vi "DriveExecute_PID_Autotune.vi"(8 "error in (no error)":errorcluster) -> (0 "error out":errorcluster)   [LabVIEW 2020]
doc: "Execute for Drie\n\nClosed control loop for drive\n\ninput: \n error in (cluster)\n\noutput:\n error out (cluster)"
uses:
  <vilib>/Rock Robotics/WPI/ThirdParty/Phoenix-LabVIEW/Motor Controller/Controls/CTRE_Phoenix_MotorControl_ControlMode.ctl
  <vilib>/Rock Robotics/WPI/ThirdParty/JAS_Junk/TrajLib/SimpleMotorFF_Calculate.vi
  <vilib>/Rock Robotics/WPI/ThirdParty/JAS_Junk/TrajLib/VI/Util_GetTime_U32.vi
  <vilib>/Rock Robotics/WPI/ThirdParty/JAS_Junk/TrajLib/PIDController_AtSetpoint.vi
  <vilib>/Rock Robotics/WPI/ThirdParty/JAS_Junk/TrajLib/PIDController_SetPIDF.vi
  <vilib>/Rock Robotics/WPI/ThirdParty/JAS_Junk/TrajLib/PIDController_SetDerivativeFilter.vi
  <vilib>/Rock Robotics/WPI/ThirdParty/JAS_Junk/TrajLib/PIDController_SetIntegratorRange.vi
  <vilib>/Rock Robotics/WPI/ThirdParty/JAS_Junk/TrajLib/PIDController_SetTolerancePandV.vi
  <vilib>/Rock Robotics/WPI/ThirdParty/JAS_Junk/TrajLib/PIDController_DisableContinousInput.vi
  <vilib>/Rock Robotics/WPI/ThirdParty/JAS_Junk/TrajLib/PIDController_EnableContinousInput.vi
  <vilib>/Rock Robotics/WPI/ThirdParty/JAS_Junk/TrajLib/PIDController_Reset.vi
  <vilib>/Rock Robotics/WPI/ThirdParty/JAS_Junk/TrajLib/PIDController_New.vi
  <vilib>/Rock Robotics/WPI/ThirdParty/JAS_Junk/TrajLib/PIDController_SetOutputLimits.vi
  <vilib>/Rock Robotics/WPI/ThirdParty/JAS_Junk/TrajLib/SlewRateLimiter_New.vi
  <vilib>/Rock Robotics/WPI/ThirdParty/JAS_Junk/TrajLib/SlewRateLimiter_Reset.vi
  <vilib>/Rock Robotics/WPI/ThirdParty/JAS_Junk/TrajLib/SlewRateLimiter_Calculate.vi
  <vilib>/Rock Robotics/WPI/ThirdParty/JAS_Junk/TrajLib/SlewRateLimiter_SetRate.vi
  <vilib>/Rock Robotics/WPI/ThirdParty/JAS_Junk/TrajLib/LinearFilter_ResetToValue.vi
  <vilib>/Rock Robotics/WPI/ThirdParty/JAS_Junk/TrajLib/LinearFilter_Calculate.vi
  <vilib>/Rock Robotics/WPI/ThirdParty/JAS_Junk/TrajLib/PIDController_NewPeriod.vi
  <vilib>/Rock Robotics/SystemInterfaces/NetworkCommunication/NetComm_UsageReport_report.vi
  <vilib>/Rock Robotics/SystemInterfaces/Utilities/FPGA_UtilitiesRead LocalTime.vi
  <vilib>/Rock Robotics/WPI/ThirdParty/JAS_Junk/TrajLib/VI/Util_GetTime_U64.vi
  DriveGlobal.vi
  <vilib>/Rock Robotics/WPI/ThirdParty/JAS_Junk/TrajLib/LinearFilter_MovingAverage.vi
  <vilib>/Rock Robotics/WPI/ThirdParty/JAS_Junk/TrajLib/LinearFilter_LowPassBW1.vi
  <vilib>/Rock Robotics/WPI/ThirdParty/JAS_Junk/TrajLib/LinearFilter_LowPassBW2.vi
  <vilib>/Rock Robotics/WPI/ThirdParty/JAS_Junk/TrajLib/LinearFilter_HighPassBW1.vi
  <vilib>/Rock Robotics/WPI/ThirdParty/JAS_Junk/TrajLib/LinearFilter_HighPassBW2.vi
  <vilib>/Rock Robotics/WPI/ThirdParty/JAS_Junk/TrajLib/Globals/Util_LibraryGlobals.vi
  <vilib>/Rock Robotics/WPI/ThirdParty/JAS_Junk/TrajLib/PIDController_AdvCalculate_FF_Sp_Pv.vi
  <vilib>/Rock Robotics/Network Tables/NT Write Value.vi
  <vilib>/Rock Robotics/Network Tables/NT Write Boolean.vi
  <vilib>/Rock Robotics/Network Tables/NT Write Number.vi
  <vilib>/Rock Robotics/WPI/ThirdParty/JAS_Junk/TrajLib/Trajectory_Library.lvlib
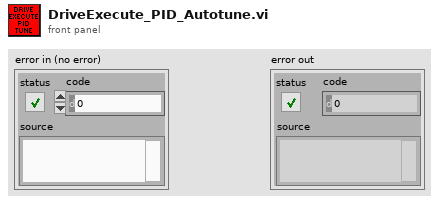
[diagram p1: front panel]
types:
  T1 = enum16{"Moving Average", "Low Pass 1st Order Butterworth", "Low Pass 2nd Order Butterworth", "High Pass 1st Order Butterworth", "High Pass 2nd Order Butterworth"}
  T2 = enum16{"Ziegler Nicols - Fast", "Ziegler Nicols - Normal", "Ziegler Nicols - Slow", "CHR regulator - 0% overshoot", "CHR regulator - 20% overshoot", "CHR servo - 0 % overshoot", "CHR servo - 20% overshoot"}
  T3 = typedef "CTRE_Phoenix_MotorControl_ControlMode.ctl" = u16
  T4 = typedef "WPI_EncoderDevRef.ctl" = cluster{"DevStatus":errorcluster, "EncoderIndex":T5, "CounterIndex":T6, "DistancePerCount":dbl, "Decoding Type":T7}
  T5 = typedef "FPGA_EncoderIdx.ctl" = enum8{"Enc 0", "Enc 1", "Enc 2", "Enc 3", "Enc 4", "Enc 5", "Enc 6", "Enc 7", "Invalid"}
  T6 = typedef "FPGA_CounterCtrSystemIndex.ctl" = enum8{"Ctr 0", "Ctr 1", "Ctr 2", "Ctr 3", "Ctr 4", "Ctr 5", "Ctr 6", "Ctr 7", "Invalid"}
  T7 = typedef "WPI_EncoderType.ctl" = enum16{"1x", "2x", "4x"}
  T8 = typedef "WPI_MotorControlDeviceRef.ctl" = cluster{"DeviceStatus":errorcluster, "Type":T9, "PWM":cluster{"PWM Channel":T10, "DeadBand":T11}, "CAN":cluster{"Device Number":u8, "SetOutput VI Ref":variant, "GetOutput VI Ref":variant, "Enable VI Ref":variant, "Disable VI Ref":variant, "Data":variant}, "Invert":bool, "DIO PWM":cluster{"PWM \"Enable\" Channel":T10, "DIOChannel":T12, "PWM Rate":dbl}}
  T9 = typedef "WPI_MotorControlType.ctl" = enum16{"PWM", "CAN", "DIO PWM"}
  T10 = typedef "FPGA_DIOPWMChannel.ctl" = enum8{"PWM 0", "PWM 1", "PWM 2", "PWM 3", "PWM 4", "PWM 5", "PWM 6", "PWM 7", "PWM 8", "PWM 9", "PWM MXP 0", "PWM MXP 1", "PWM MXP 2", "PWM MXP 3", "PWM MXP 4", "PWM MXP 5", "PWM MXP 6", "PWM MXP 7", "PWM MXP 8", "PWM MXP 9", "Invalid"}
  T11 = typedef "WPI_PWMDeadband.ctl" = cluster{"Name":string, "maxPositivePwm":i32, "minPositivePwm":i32, "centerPwm":i32, "maxNegativePwm":i32, "minNegativePwm":i32, "angularRange":u16}
  T12 = typedef "FPGA_DIOChannel.ctl" = enum8{"DIO 0", "DIO 1", "DIO 2", "DIO 3", "DIO 4", "DIO 5", "DIO 6", "DIO 7", "DIO 8", "DIO 9", "DIO MXP 0", "DIO MXP 1", "DIO MXP 2", "DIO MXP 3", "DIO MXP 4", "DIO MXP 5", "DIO MXP 6", "DIO MXP 7", "DIO MXP 8", "DIO MXP 9", "DIO MXP 10", "DIO MXP 11", "DIO MXP 12", "DIO MXP 13", "DIO MXP 14", "DIO MXP 15", "SPI Port CS1", "SPI Port CS2", "SPI Port CS3", "SPI Port MISO", "SPI Port MOSI", "Invalid"}
  T13 = typedef "ADIS16470 Device Reference.ctl" = cluster{"DevStatus":errorcluster, "Hardware Config":T14, "Calibration Complete":refnum<notifier>, "Status Reference":refnum<data-value>, "Data Reference":refnum<data-value>, "Sychronous Process VI":T17, "Cmd FIFO":refnum<k33>, "Source":T18, "Data FIFO":refnum<k33>, "Calibration Time (ms)":u32, "Data Reference":refnum<data-value>}
  T14 = typedef "ADIS16470 Hardware Configuration.ctl" = cluster{"SPI Clock Rate (Hz)":dbl, "IMU SPI Mode (3)":T15, "IMU Reset Pin":T12, "IMU SPI Bus":T16, "IMU Data Ready Pin":T12, "Stall Config":cluster{"Pow2BytesPerRead":u8, "StallTicks":u16, "CsToSclkTicks":u8}}
  T15 = typedef "WPI_SPIMode.ctl" = enum16{"Mode 0 (Clk Idle Low,Sample on Leading)", "Mode 1 (Clk Idle Low,Sample on Trailing)", "Mode 2 (Clk Idle High,Sample on Leading)", "Mode 3 (Clk Idle High,Sample on Trailing)"}
  T16 = typedef "spi_bus.ctl" = enum16{"SPI On-Board, CS0", "SPI On-Board, CS1", "SPI On-Board, CS2", "SPI On-Board, CS3", "SPI MXP", "Invalid"}
  T17 = typedef "ADIS16470 Process.ctl" = refnum<vi>
  T18 = typedef "FPGA_CounterEncoderSourceConvertionLVSourceType.ctl" = cluster{"DevStatus":errorcluster, "AnalogTriggerMode?":bool, "DigitalMode":cluster{"DIO Channel":T19}, "AnalogTriggerMode":cluster{"AnalogTriggerIndex":T20, "OutputType":T21}}
  T19 = typedef "FPGA_DIODigitalSourceChannel.ctl" = enum8{"DIO 0", "DIO 1", "DIO 2", "DIO 3", "DIO 4", "DIO 5", "DIO 6", "DIO 7", "DIO 8", "DIO 9", "DIO MXP 0", "DIO MXP 1", "DIO MXP 2", "DIO MXP 3", "DIO MXP 4", "DIO MXP 5", "DIO MXP 6", "DIO MXP 7", "DIO MXP 8", "DIO MXP 9", "DIO MXP 10", "DIO MXP 11", "DIO MXP 12", "DIO MXP 13", "DIO MXP 14", "DIO MXP 15", "SPI Port CS1", "SPI Port CS2", "SPI Port CS3", "SPI Port MISO", "SPI Port MOSI", "Disabled"}
  T20 = typedef "FPGA_AnalogTriggerIndex.ctl" = enum8{"Trig 0", "Trig 1", "Trig 2", "Trig 3", "Trig 4", "Trig 5", "Trig 6", "Trig 7", "Invalid"}
  T21 = typedef "FPGA_AnalogTriggerOutType.ctl" = enum16{"InWindow", "TriggerState", "Rising", "Falling"}
  T22 = typedef "ADIS16470 Data.ctl" = cluster{"XAngle":dbl, "YAngle":dbl, "ZAngle":dbl}
  T23 = typedef "Trajectory_Library.lvlib/SIMPLE_MOTOR_FF.ctl" = cluster{"Ks":dbl, "Kv":dbl, "Ka":dbl, "KnInv":dbl}
  T24 = typedef "Trajectory_Library.lvlib/PID_ADV_LIMITS.ctl" = cluster{"MaxInput":dbl, "MinInput":dbl, "Continuous":bool, "MaxOutput":dbl, "MinOutput":dbl}
  T25 = typedef "Trajectory_Library.lvlib/PID_ADV_TUNING.ctl" = cluster{"Kf":dbl, "Kp":dbl, "Ki":dbl, "Kd":dbl, "MaximumIntegral":dbl, "MinimumIntegral":dbl, "Filter Derivative":bool}
  T26 = cluster{"Controller Constant Type":enum16{"Ziegler Nicols - Fast", "Ziegler Nicols - Normal", "Ziegler Nicols - Slow", "CHR regulator - 0% overshoot", "CHR regulator - 20% overshoot", "CHR servo - 0 % overshoot", "CHR servo - 20% overshoot"}, "Type of Controller":enum16{"P", "PI", "PID"}, "CO Offset":dbl, "Kn":dbl, "Tuning Tolerance":dbl, "Plant Tolerance":dbl, "Newest Avg Time ":i32, "Long Ave Time":i32}
  T27 = cluster{"Plant Gain (K)":dbl, "Time Constant (T)":dbl, "Dead Time (L)":dbl, "stimulus operating point":dbl, "response operating point":dbl}
  T28 = cluster{"proportional gain (Kp)":dbl, "integral time (Ki / Sec)":dbl, "derivative time (Kd /Sec)":dbl}
  T29 = cluster{"Const Done":bool, "Plant Done":bool, "PV Std Dev":dbl, "CO Std Dev":dbl}
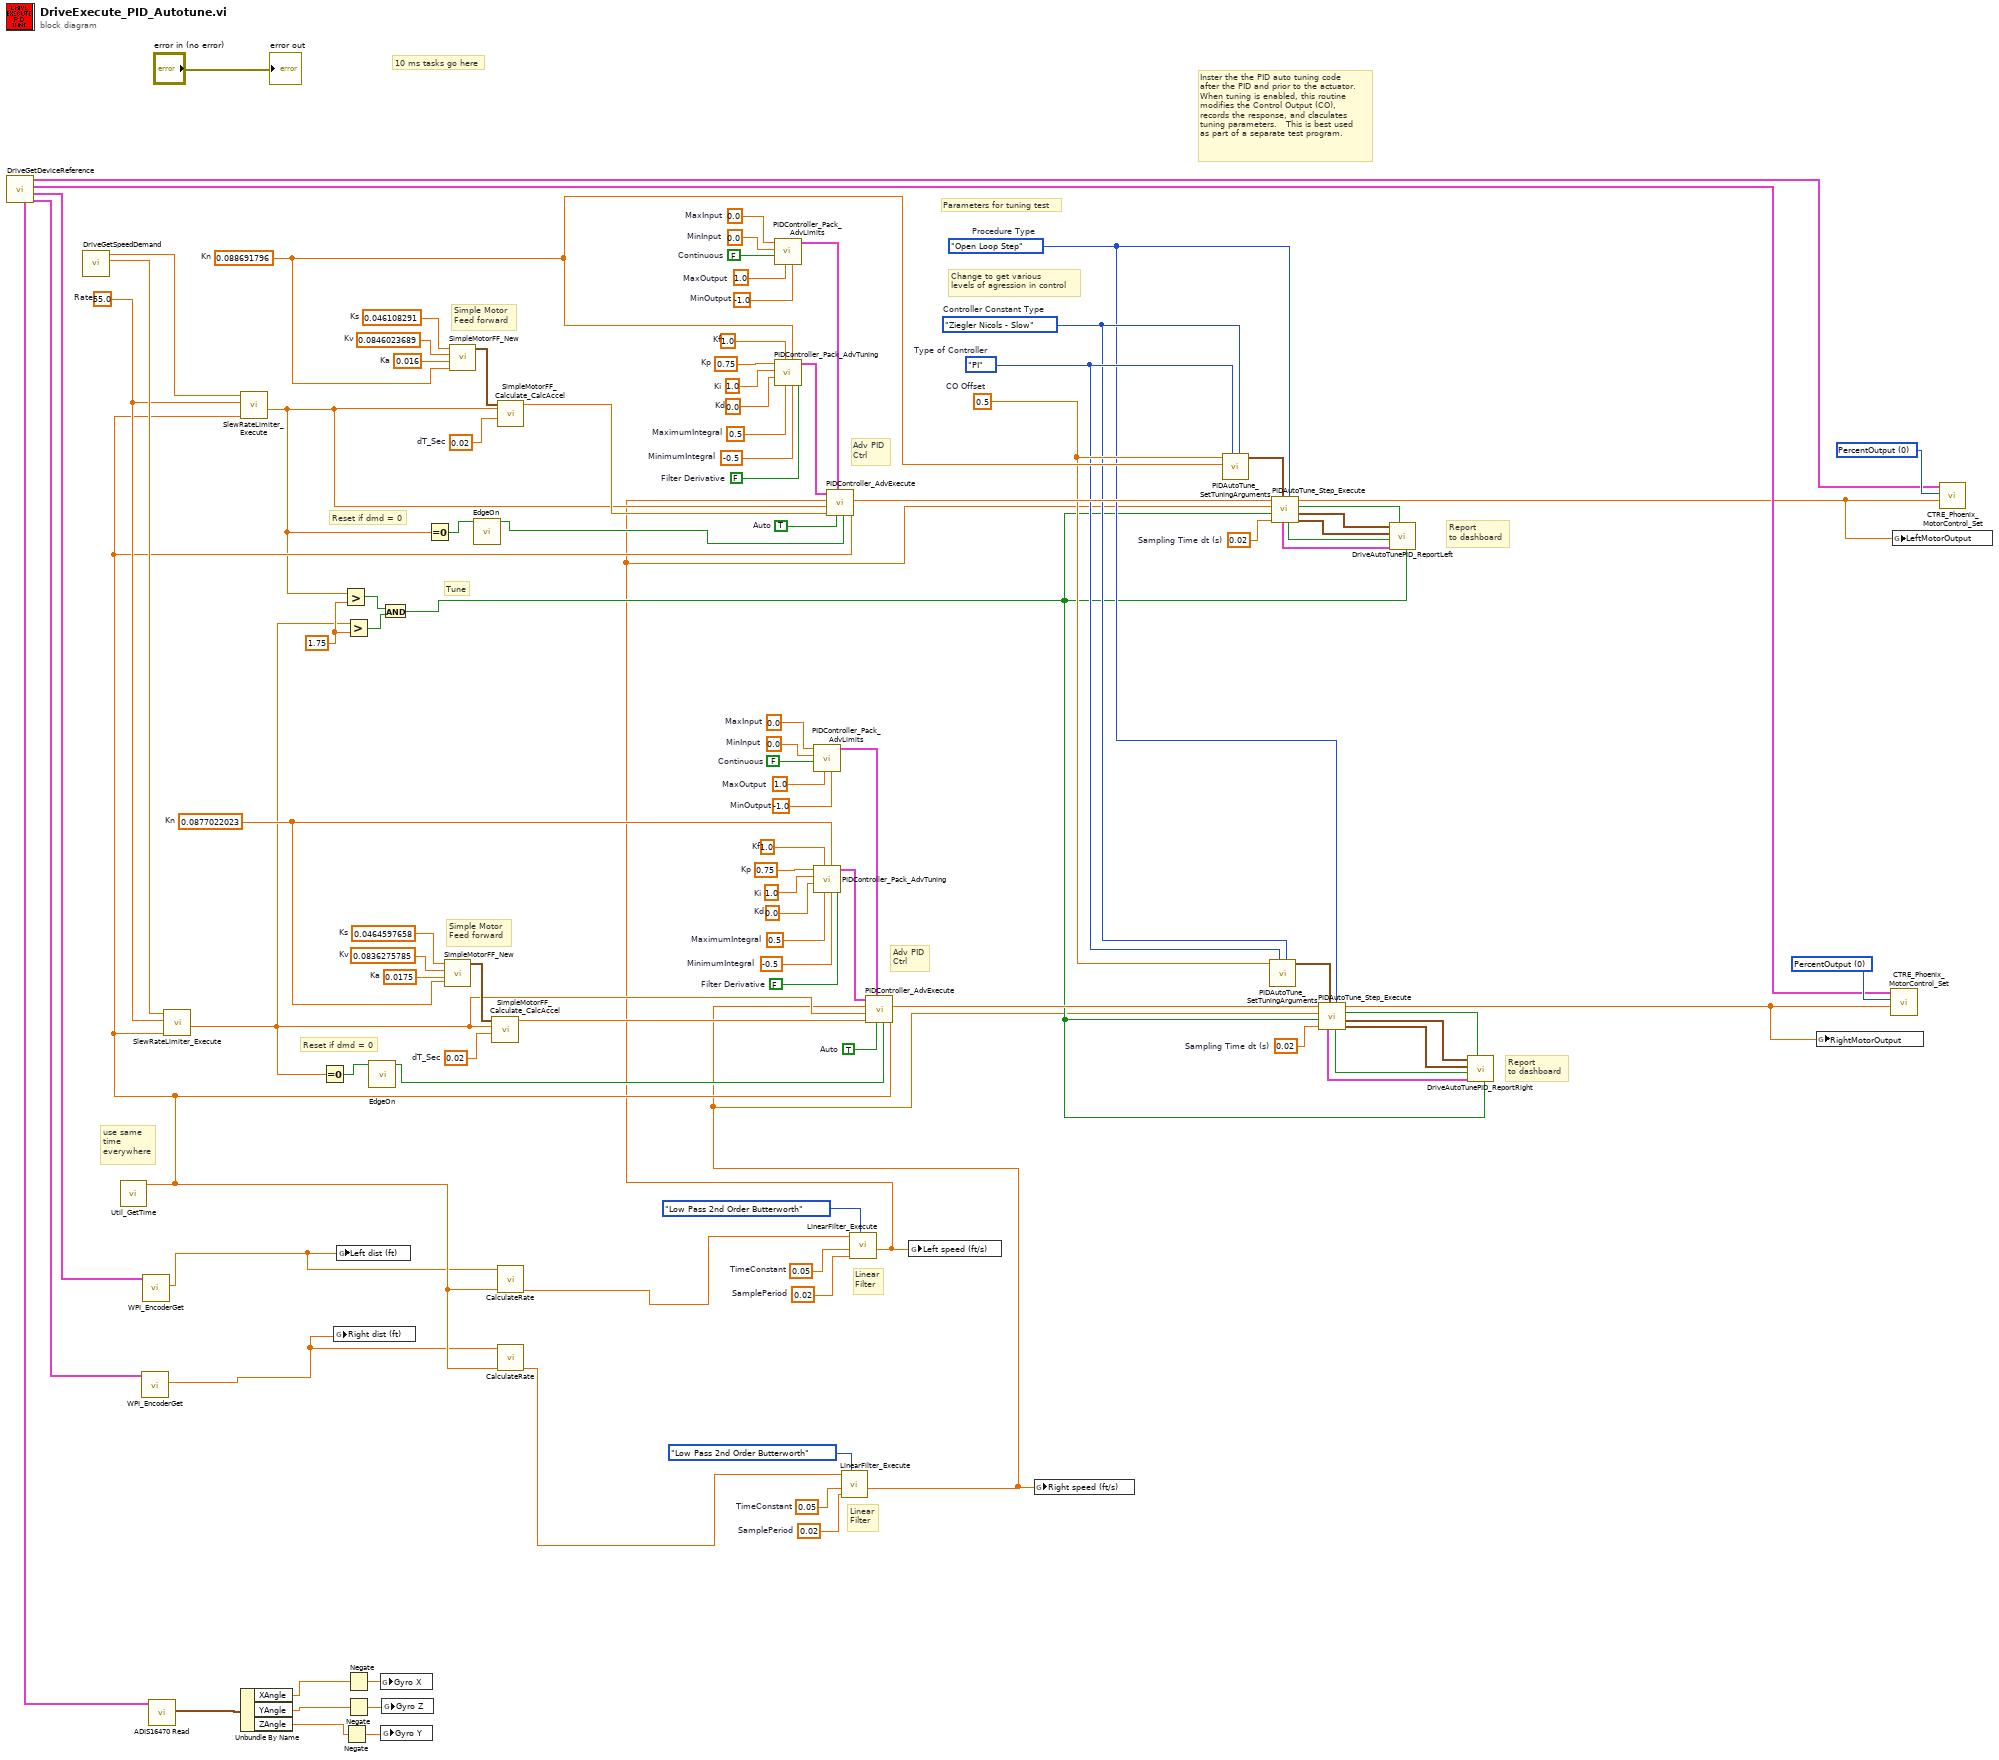
[diagram p0: block diagram]
diagram:
  w11 = 0.02  # SamplePeriod
  w10 = 0.05  # TimeConstant
  w14 = 0.02  # SamplePeriod
  w13 = 0.05  # TimeConstant
  w37 = enum16{"Open Loop Step", "Closed Loop Step"}."Open Loop Step"  # Procedure Type
  w38 = T2."Ziegler Nicols - Slow"  # Controller Constant Type
  w39 = enum16{"P", "PI", "PID"}."PI"  # Type of Controller
  w40 = 0.5  # CO Offset
  w35 = 1.75
  w44 = 0.02  # Sampling Time dt (s)
  w49 = 0.02  # Sampling Time dt (s)
  w50 = 55.0  # Rate
  w64 = TRUE  # Auto
  w19 = TRUE  # Auto
  w65 = 0.0877022023  # Kn
  w79 = 0.75  # Kp
  w78 = 1.0  # Ki
  w77 = 0.0  # Kd
  w76 = 1.0  # Kf
  w75 = 0.5  # MaximumIntegral
  w74 = -0.5  # MinimumIntegral
  w73 = FALSE  # Filter Derivative
  w71 = 0.0  # MinInput
  w70 = FALSE  # Continuous
  w69 = 1.0  # MaxOutput
  w72 = -1.0  # MinOutput
  w68 = 0.0  # MaxInput
  w45 = 0.088691796  # Kn
  w92 = 0.75  # Kp
  w51 = 1.0  # Ki
  w91 = 0.0  # Kd
  w90 = 1.0  # Kf
  w89 = 0.5  # MaximumIntegral
  w88 = -0.5  # MinimumIntegral
  w87 = FALSE  # Filter Derivative
  w85 = 0.0  # MinInput
  w84 = FALSE  # Continuous
  w83 = 1.0  # MaxOutput
  w86 = -1.0  # MinOutput
  w82 = 0.0  # MaxInput
  w97 = 0.02  # dT_Sec
  w95 = 0.0464597658  # Ks
  w94 = 0.0836275785  # Kv
  w93 = 0.0175  # Ka
  w102 = 0.02  # dT_Sec
  w100 = 0.046108291  # Ks
  w99 = 0.0846023689  # Kv
  w98 = 0.016  # Ka
  w106 = T3 0 items=["PercentOutput"=0, "Position"=1, "Velocity"=2, "Current"=3, "Follower"=5, "MotionProfile"=6, "MotionMagic"=7, "MotionProfileArc"=10, "Disabled"=15] ("Control Mode")
  w107 = T3 0 items=["PercentOutput"=0, "Position"=1, "Velocity"=2, "Current"=3, "Follower"=5, "MotionProfile"=6, "MotionMagic"=7, "MotionProfileArc"=10, "Disabled"=15] ("Control Mode")
  # "Linear\nFilter"
  # "Linear\nFilter"
  # "Reset if dmd = 0"
  # "Reset if dmd = 0"
  # "Report \nto dashboard"
  # "Report \nto dashboard"
  # "Change to get various\nlevels of agression in control"
  # "Parameters for tuning test"
  # "Tune"
  # "Inster the the PID auto tuning code\nafter the PID and prior to the actuator.\nWhen tuning is enabled, this routine\nmodifies the Control Output (CO), \nrecords the response, and claculates\ntuning parameters.   This is best used\nas part of a separate test program."
  # "use same\ntime\neverywhere"
  # "Adv PID\nCtrl"
  # "Adv PID\nCtrl"
  # "Simple Motor\nFeed forward"
  # "Simple Motor\nFeed forward"
  # "10 ms tasks go here"
  n1 = call "DriveGetDeviceReference.vi"() -> ("RightDriveEncoder"=w5:T4, "LeftDriveEncoder"=w6:T4, "RightDriveTrain"=w60:T8, "LeftDriveTrain"=w61:T8, "Gryo"=w103:T13)  [unwired: 7 in]
  n2 = call "DriveGetSpeedDemand.vi"() -> ("RSpeedDemand (ft/s)"=w58:dbl, "LSpeedDemand (ft/s)"=w59:dbl)  [unwired: 10 in]
  n3 = call <vilib>:"Util_GetTime.vi"() -> ("FPGA_Time_Seconds"=w41:dbl)  [unwired: 9 in, 2 out]
  n4 = call <vilib>:"WPI_EncoderGet.vi"("EncoderDevRef"=w5) -> ("Distance"=w3:dbl)  [unwired: 5 in, 5 out]
  n5 = call <vilib>:"WPI_EncoderGet.vi"("EncoderDevRef"=w6) -> ("Distance"=w4:dbl)  [unwired: 5 in, 5 out]
  n6 = call <vilib>:"ADIS16470 Read.vi"("ADIS16470DevRef"=w103) -> ("ADIS16470 Value"=w104:T22)  [unwired: 7 in, 3 out]
  n7 = call <vilib>:"SlewRateLimiter_Execute.vi"("Time"=w41, "PositiveRate"=w50, "Input"=w58) -> ("Output"=w16:dbl)  [unwired: 7 in, 1 out]
  n8 = call <vilib>:"SlewRateLimiter_Execute.vi"("Time"=w41, "PositiveRate"=w50, "Input"=w59) -> ("Output"=w21:dbl)  [unwired: 7 in, 1 out]
  n9 = Unbundle By Name(w104) -> ("XAngle"=w52:dbl, "YAngle"=w54:dbl, "ZAngle"=w53:dbl)
  n10 = Equal To 0?(x=w16) -> (x = 0?=w17:bool)
  n11 = global write "DriveGlobal.vi" "Right dist (ft)"(w3) -> ()
  n12 = global write "DriveGlobal.vi" "Left dist (ft)"(w4) -> ()
  n13 = Greater?(x=w21, y=w35) -> (0:w34:bool)
  n14 = Negate(x=w53) -> (-x=w56:dbl)
  n15 = Greater?(x=w16, y=w35) -> (0:w33:bool)
  n16 = Negate(x=w52) -> (-x=w57:dbl)
  n17 = Negate(x=w54) -> (-x=w55:dbl)
  n18 = call "EdgeOn.vi"("Current State"=w17) -> ("Edge On Found"=w15:bool)  [unwired: 10 in]
  n19 = global write "DriveGlobal.vi" "Gyro X"(w57) -> ()
  n20 = global write "DriveGlobal.vi" "Gyro Y"(w56) -> ()
  n21 = global write "DriveGlobal.vi" "Gyro Z"(w55) -> ()
  n22 = And(x=w34, y=w33) -> (x .and. y?=w22:bool)
  n23 = Equal To 0?(x=w21) -> (x = 0?=w20:bool)
  n24 = call <vilib>:"SimpleMotorFF_New.vi"("Kn"=w65, "Ka"=w93, "Kv"=w94, "Ks"=w95) -> ("SIMPLE_MOTOR_FF"=w96:T23)  [unwired: 7 in]
  n25 = call <vilib>:"SimpleMotorFF_New.vi"("Kn"=w45, "Ka"=w98, "Kv"=w99, "Ks"=w100) -> ("SIMPLE_MOTOR_FF"=w101:T23)  [unwired: 7 in]
  n26 = call "EdgeOn.vi"("Current State"=w20) -> ("Edge On Found"=w18:bool)  [unwired: 10 in]
  n27 = call <vilib>:"SimpleMotorFF_Calculate_CalcAccel.vi"("dT_Sec"=w97, "VelSp"=w16, "SIMPLE_MOTOR_FF"=w96) -> ("FeedForward"=w62:dbl)  [unwired: 8 in]
  n28 = call <vilib>:"SimpleMotorFF_Calculate_CalcAccel.vi"("dT_Sec"=w102, "VelSp"=w21, "SIMPLE_MOTOR_FF"=w101) -> ("FeedForward"=w63:dbl)  [unwired: 8 in]
  n29 = call "CalculateRate.vi"("Time (s)"=w41, "Distance (units)"=w4) -> ("Rate (units/s)"=w1:dbl)  [unwired: 9 in]
  n30 = call "CalculateRate.vi"("Time (s)"=w41, "Distance (units)"=w3) -> ("Rate (units/s)"=w2:dbl)  [unwired: 9 in]
  n31 = call <vilib>:"PIDController_Pack_AdvLimits.vi"("MinOutput"=w86, "MaxOutput"=w83, "Continuous"=w84, "MinInput"=w85, "MaxInput"=w82) -> ("Adv PID Limits"=w80:T24)  [unwired: 6 in]
  n32 = call <vilib>:"PIDController_Pack_AdvTuning.vi"("Filter Derivative"=w87, "MinimumIntegral"=w88, "Kn"=w45, "MaximumIntegral"=w89, "Kf"=w90, "Kd"=w91, "Ki"=w51, "Kp"=w92) -> ("Adv PID Tuning"=w81:T25)  [unwired: 3 in]
  n33 = call <vilib>:"PIDController_Pack_AdvLimits.vi"("MinOutput"=w72, "MaxOutput"=w69, "Continuous"=w70, "MinInput"=w71, "MaxInput"=w68) -> ("Adv PID Limits"=w66:T24)  [unwired: 6 in]
  n34 = call <vilib>:"PIDController_Pack_AdvTuning.vi"("Filter Derivative"=w73, "MinimumIntegral"=w74, "Kn"=w65, "MaximumIntegral"=w75, "Kf"=w76, "Kd"=w77, "Ki"=w78, "Kp"=w79) -> ("Adv PID Tuning"=w67:T25)  [unwired: 3 in]
  n35 = call <vilib>:"LinearFilter_Execute.vi"("Filter Type"=T1."Low Pass 2nd Order Butterworth", "SamplePeriod"=w11, "TimeConstant"=w10, "Input"=w2) -> ("Output"=w7:dbl)  [unwired: 6 in, 1 out]
  n36 = call <vilib>:"LinearFilter_Execute.vi"("Filter Type"=T1."Low Pass 2nd Order Butterworth", "SamplePeriod"=w14, "TimeConstant"=w13, "Input"=w1) -> ("Output"=w8:dbl)  [unwired: 6 in, 1 out]
  n37 = call <vilib>:"PIDController_AdvExecute.vi"("Time"=w41, "Reset"=w18, "Auto"=w19, "Adv PID Limits"=w80, "FF-FeedForward"=w63, "SP-SetPoint"=w21, "PV-Measurement"=w8, "Adv PID Tuning"=w81) -> ("CO-ControlOutput"=w47:dbl)  [unwired: 1 in, 2 out]
  n38 = call <vilib>:"PIDController_AdvExecute.vi"("Time"=w41, "Reset"=w15, "Auto"=w64, "Adv PID Limits"=w66, "FF-FeedForward"=w62, "SP-SetPoint"=w16, "PV-Measurement"=w7, "Adv PID Tuning"=w67) -> ("CO-ControlOutput"=w42:dbl)  [unwired: 1 in, 2 out]
  n39 = global write "DriveGlobal.vi" "Left speed (ft/s)"(w8) -> ()
  n40 = global write "DriveGlobal.vi" "Right speed (ft/s)"(w7) -> ()
  n41 = call <vilib>:"PIDAutoTune_SetTuningArguments.vi"("Controller Constant Type"=w38, "Type of Controller"=w39, "Kn"=w45, "CO Offset"=w40) -> ("Configuration Parameters"=w48:T26)  [unwired: 7 in]
  n42 = call <vilib>:"PIDAutoTune_SetTuningArguments.vi"("Controller Constant Type"=w38, "Type of Controller"=w39, "CO Offset"=w40) -> ("Configuration Parameters"=w43:T26)  [unwired: 8 in]
  n43 = call <vilib>:"PIDAutoTune_Step_Execute.vi"("Procedure Type"=w37, "Configuration Parameters"=w48, "Sampling Time dt (s)"=w49, "Tune"=w22, "Measurement  (PV)"=w8, "Control Output (Co)"=w47) -> ("Plant and Test Data"=w31:T27, "New Tuning Parameters"=w32:T28, "Tuning Done"=w30:bool, "Adj CO"=w46:dbl, "Error Occured"=w29:bool, "Diagnostic Info"=w28:T29)
  n44 = call <vilib>:"PIDAutoTune_Step_Execute.vi"("Procedure Type"=w37, "Configuration Parameters"=w43, "Sampling Time dt (s)"=w44, "Tune"=w22, "Measurement  (PV)"=w7, "Control Output (Co)"=w42) -> ("Plant and Test Data"=w25:T27, "New Tuning Parameters"=w26:T28, "Tuning Done"=w27:bool, "Adj CO"=w36:dbl, "Error Occured"=w24:bool, "Diagnostic Info"=w23:T29)
  n45 = call "DriveAutoTunePID_ReportLeft.vi"("Tuning in Progress"=w22, "Tuning Done in"=w30, "Diagnostic Info in"=w28, "Error Occured in"=w29, "Plant and Test Data in"=w31, "New Tuning Parameters in"=w32) -> ()  [unwired: 6 in]
  n46 = call "DriveAutoTunePID_ReportRight.vi"("Tuning in Progress"=w22, "Tuning Done in"=w27, "Diagnostic Info in"=w23, "Error Occured in"=w24, "Plant and Test Data in"=w25, "New Tuning Parameters in"=w26) -> ()  [unwired: 6 in]
  n47 = global write "DriveGlobal.vi" "RightMotorOutput"(w36) -> ()
  n48 = call <vilib>:"CTRE_Phoenix_MotorControl_Set.vi"("Output"=w36, "Control Mode"=w106, "PhoenixMotorControlDevRef"=w60) -> ()  [unwired: 7 in, 2 out]
  n49 = global write "DriveGlobal.vi" "LeftMotorOutput"(w46) -> ()
  n50 = call <vilib>:"CTRE_Phoenix_MotorControl_Set.vi"("Output"=w46, "Control Mode"=w107, "PhoenixMotorControlDevRef"=w61) -> ()  [unwired: 7 in, 2 out]
  "error out" <- "error in (no error)"
